vi "keithley2400 measure current.vi"(8 "error in (no error)":errorcluster, 11 "VISA resource name":refnum<visa-resource-name>) -> (0 "error out":errorcluster, 3 "Current mA":dbl)   [LabVIEW 2024]
doc: "This example shows how to configure a measurement and take a reading."
panel:
  # "(c) 2006 National Instruments.  ALL RIGHTS RESERVED."
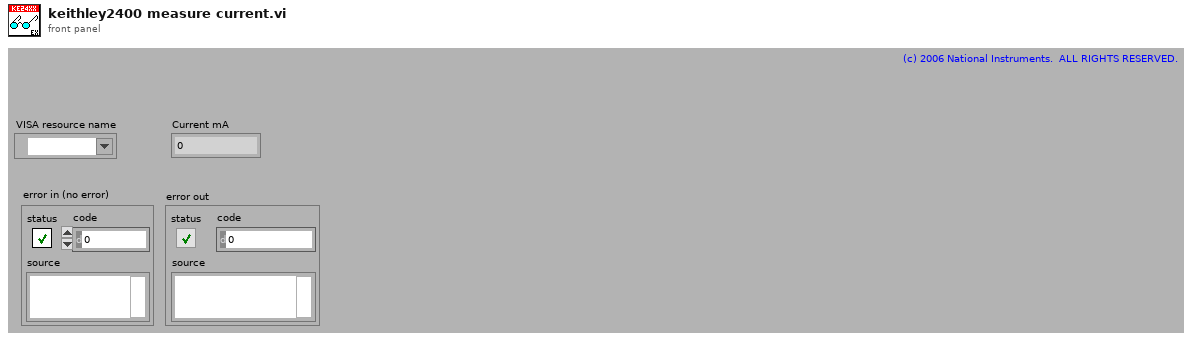
[diagram p1: front panel]
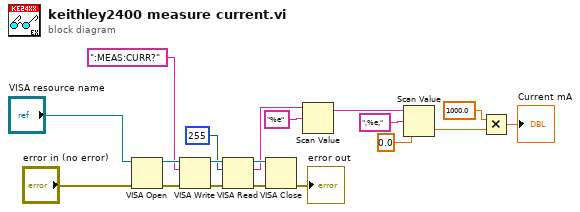
[diagram p0: block diagram]
diagram:
  n1 = VISA Open(error in (no error)="error in (no error)", VISA resource name="VISA resource name") -> (VISA resource name=w16:refnum<visa-resource-name>, error out=w14:errorcluster)  [unwired: 3 in]
  n2 = VISA Write(VISA resource name=w16, write buffer=":MEAS:CURR?", error in (no error)=w14) -> (VISA resource name out=w18:refnum<visa-resource-name>, error out=w19:errorcluster)  [unwired: 1 out]
  n3 = VISA Read(VISA resource name=w18, byte count=u32 255, error in (no error)=w19) -> (VISA resource name out=w11:refnum<visa-resource-name>, read buffer=w6:string, error out=w12:errorcluster)  [unwired: 1 out]
  n4 = VISA Close(VISA resource name=w11, error in (no error)=w12) -> (error out=→"error out":errorcluster)
  n5 = Scan Value(string=w6, format string="%e") -> (output string=w4:string)  [unwired: 1 in, 1 out]
  n6 = Scan Value(string=w4, format string=",%e,", default (0 dbl)=0.0) -> (value=w2:dbl)  [unwired: 1 out]
  n7 = Multiply(x=1000.0, y=w2) -> (x*y=→"Current mA":dbl)
